vi "Display Unopenable Message.vi"(8 "error in (no error)":errorcluster, 10 "SubPanel":refnum<vi>, 11 "Standard VI Type in":refnum<class "Standard VI Type.lvclass">) -> (0 "error out":errorcluster, 3 "Standard VI Type out":refnum<class "Standard VI Type.lvclass">)   [LabVIEW 2020, in "Peek Window.lvlib" / "Standard VI Type.lvclass"]
uses:
  Missing VI Type/Missing VI Type.lvclass/Missing VI Type.ctl
  Standard VI Type.lvclass
  Standard VI Type.lvclass/Standard VI Type.ctl
  Not Openable VI Message.vi
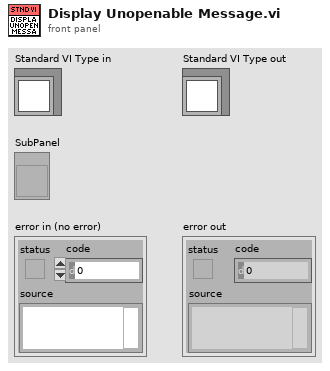
[diagram p1: front panel]
types:
  T1 = enum8{"Enabled", "Disabled", "Disabled and Grayed Out"}
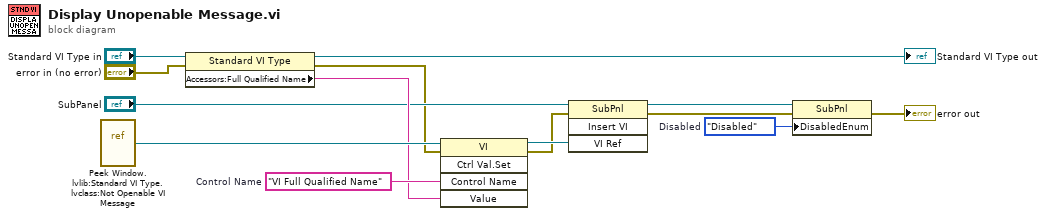
[diagram p0: block diagram]
diagram:
  w5 = T1."Disabled"  # Disabled
  w13 = "VI Full Qualified Name"  # Control Name
  n1 = vi-ref "Peek Window.lvlib:Standard VI Type.lvclass:Not Openable VI Message.vi"() -> (w12:refnum<vi>)
  n2 = property class="Standard VI Type"(reference="Standard VI Type in", error in="error in (no error)") -> (reference out=→"Standard VI Type out":refnum<class "Standard VI Type.lvclass">, error out=w3:errorcluster, "Accessors:Full Qualified Name"=w11:string)
  n3 = invoke class="VI" method="Ctrl Val.Set"(reference=w12, error in=w3, "Control Name"=w13, "Value"=w11) -> (reference out=w2:refnum<vi>, error out=w1:errorcluster)  [unwired: 1 in, 3 out]
  n4 = invoke class="SubPnl" method="Insert VI"(reference="SubPanel", error in=w1, "VI Ref"=w2) -> (reference out=w7:refnum<vi>, error out=w8:errorcluster)  [unwired: 1 in, 2 out]
  n5 = property class="SubPnl"(reference=w7, error in=w8, "DisabledEnum"=w5) -> (error out=→"error out":errorcluster)  [unwired: 1 out]
